vi "calculateHistogram.vi"(8 "error in (no error)":errorcluster, 11 "ax5 in":refnum<class "ax5.lvclass">) -> (0 "error out":errorcluster, 2 "tempHistogram":T1 {"Standard  Variation" format="%.2f"; "Mean Value" format="%.2f"; "Interval Width" format="%.2f"; "Starting Value" format="%.2f"; "Maximal Value" format="%.2f"; "Minimal Value" format="%.2f"}, 3 "ax5 out":refnum<class "ax5.lvclass">)   [LabVIEW 2017, in "ax5.lvclass"]
uses:
  ax5.lvclass
  \\psf\Home/Desktop/Elkhorn Test/Elkhorn Test/JSONRPC Server Framework Examples/builds/JSON RPC over TCP/RT CompactRIO Target/My Source Distribution/home/lvuser/natinst/bin/methods/camera.lvclass
  <vilib>/vision/NI_Vision_Development_Module.lvlib
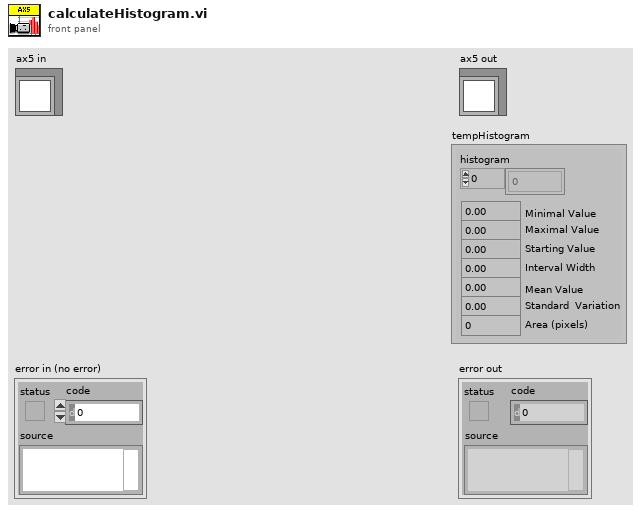
[diagram p1: front panel]
types:
  T1 = cluster{"histogram":u32[], "Minimal Value":sgl, "Maximal Value":sgl, "Starting Value":sgl, "Interval Width":sgl, "Mean Value":sgl, "Standard  Variation":sgl, "Area (pixels)":i32}
  T2 = typedef "IMAQ Image.ctl" = refnum<image>
  T3 = cluster{"histogram":dbl[], "Minimal Value":dbl, "Maximal Value":dbl, "Starting Value":dbl, "Interval Width":dbl, "Mean Value":dbl, "Standard  Variation":dbl, "Area (pixels)":dbl}
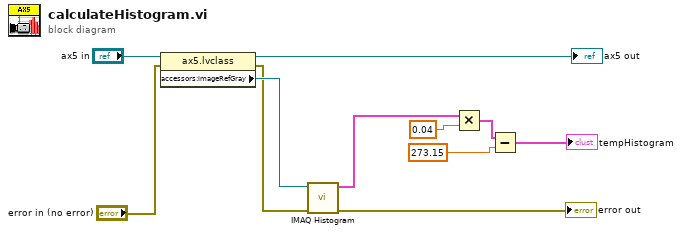
[diagram p0: block diagram]
diagram:
  n1 = property class="ax5.lvclass"(reference="ax5 in", error in="error in (no error)") -> (reference out=→"ax5 out":refnum<class "ax5.lvclass">, error out=w7:errorcluster, "accessors:imageRefGray"=w9:T2)
  n2 = call "IMAQ Histogram"("error in (no error)"=w7, "Image"=w9) -> ("error out"=→"error out":errorcluster, "Histogram Report"=w2:T1)  [unwired: 8 in]
  n3 = Multiply(x=w2, y=0.04) -> (x*y=w4:T3)
  n4 = Subtract(x=w4, y=273.15) -> (x-y=→"tempHistogram":T3)
